vi "Get Wavelength.vi"(8 "error in (no error)":errorcluster, 11 "Topas4 in":refnum<class "Topas4.lvclass">) -> (0 "error out":errorcluster, 2 "Wavelength":dbl, 3 "Topas4 out":refnum<class "Topas4.lvclass">)   [LabVIEW 2020, in "Topas4.lvclass"]
uses:
  Topas4.lvclass
  Topas4.lvclass/Topas4.ctl
  Topas4-LabVIEW-Driver/Library/Topas4.lvlib
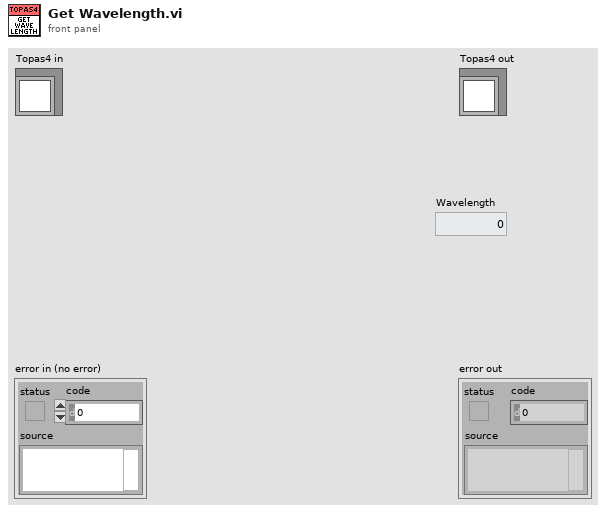
[diagram p1: front panel]
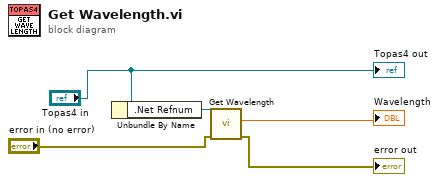
[diagram p0: block diagram]
diagram:
  n1 = Unbundle By Name("Topas4 in") -> (".Net Refnum"=w4:refnum<k24>)
  n2 = call "Get Wavelength.vi"("error in"="error in (no error)", "reference"=w4) -> ("error out"=→"error out":errorcluster, "GetOutputWavelength"=→"Wavelength":dbl)  [unwired: 7 in, 1 out]
  "Topas4 out" <- "Topas4 in"
